vi "U8 to Serial Data.vi"(7 "Parity Bit?":bool=TRUE, 10 "Parity Count In":u8, 11 "Read/Write Data":T2 {"Data" format="%.0x"}) -> (2 "Parity Out":u8, 3 "Data Values":T3[](array[typedef]))   [LabVIEW 2013]
doc: "This VI converts a U8 into an array of MIPI samples (MSB first). In order to use this Data to Array must be called."
uses:
  Ctrls/BitStates.ctl
  Ctrls/Read_Write_Data.ctl
  Ctrls/BitType.ctl
panel:
  out "Bit Types":T1[](array[typedef])
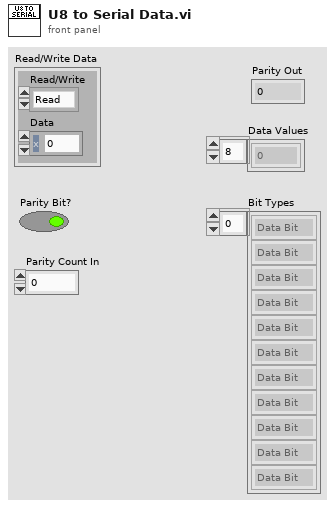
[diagram p1: front panel]
types:
  T1 = typedef "BitType.ctl" = enum16{"Data Bit", "Parity Bit"}
  T2 = typedef "Read_Write_Data.ctl" = cluster{"Data":u8, "Read/Write":enum16{"Read", "Write"}}
  T3 = typedef "BitStates.ctl" = enum16{"0", "1", "Z", "L", "H", "X", "Toggle"}
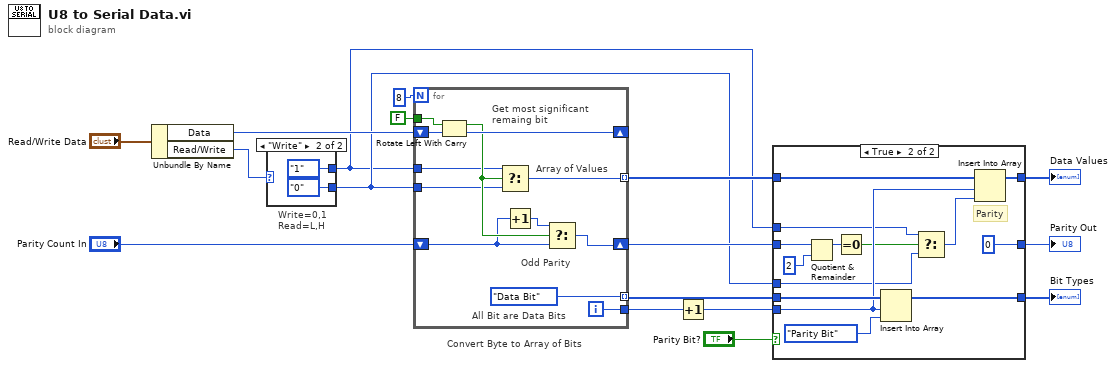
[diagram p0: block diagram]
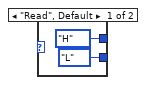
[diagram p2: hidden frame]
diagram:
  # "Convert Byte to Array of Bits"
  # "Write=0,1\nRead=L,H"
  n1 = Unbundle By Name("Read/Write Data") -> ("Data"=w16:u8, "Read/Write"=w8:enum16{"Read", "Write"})
  n2 = case shown="\"Write\"" w8 {
    tunnel: [BitStates."L" ("f") BitStates."0" ("f")] -> w2
    tunnel: [BitStates."H" ("Data Value") BitStates."1" ("Data Value")] -> w1
    frame "Read", Default {
    }
    frame "Write" {
    }
  }
  n3 = for {
    N: 8 -> [_]
    tunnel: FALSE ("carry") -> [w31]
    tunnel: [w30] -> w9 mode=indexing
    shift-right: [w32] -> _
    shift-left: w16 -> [w33]
    shift-right: [w26] -> w7
    shift-left: "Parity Count In" -> [w27]
    tunnel: w2 -> [w25]
    tunnel: w1 -> [w24]
    tunnel: [BitType."Data Bit" ("Bit Type")] -> w6 mode=indexing
    tunnel: [w22] -> w5
    i -> [w22]
    # "All Bit are Data Bits"
    # "Odd Parity"
    # "Array of Values"
    # "Get most significant remaing bit"
    n4 = Rotate Left With Carry(2:w33, 3:w31) -> (0:w32:u8, 1:w29:bool)
    n5 = Select(t=w24, s=w29, f=w25) -> (s? t:f=w30:T3)
    n6 = Increment(x=w27) -> (x+1=w28:u8)
    n7 = Select(t=w28, s=w29, f=w27) -> (s? t:f=w26:u8)
  }
  n8 = Increment(x=w5) -> (x+1=w3:i32)
  n9 = case shown="True" "Parity Bit?" {
    tunnel: w9 -> [w36 w50]
    tunnel: [w36 w49] -> w17
    tunnel: w7 -> [w35 w37]
    tunnel: [w35 u8 0 ("Parity Count In")] -> w12
    tunnel: w6 -> [w34 w46]
    tunnel: [w34 w45] -> w4
    tunnel: w3 -> [_ w43]
    tunnel: w1 -> [_ w39]
    tunnel: w2 -> [_ w38]
    frame False {
    }
    frame True {
      # "Parity"
      n10 = Quotient & Remainder(x=w37, y=u8 2) -> (x-y*floor(x/y)=w40:u8)  [unwired: 1 out]
      n11 = Equal To 0?(x=w40) -> (x = 0?=w41:bool)
      n12 = Insert Into Array(array=w46, index=w43, new element=BitType."Parity Bit" ("Bit Type")) -> (w45:T1[])
      n13 = Select(t=w39, s=w41, f=w38) -> (s? t:f=w42:T3)
      n14 = Insert Into Array(array=w50, index=w43, new element=w42) -> (w49:T3[])
    }
  }
  "Data Values" <- w17
  "Parity Out" <- w12
  "Bit Types" <- w4
